vi "Arm Globals.vi"() -> ()   [LabVIEW 2012]
panel:
  in  "Arm Def Speed":dbl=0.5
  in  "Arm Dump Speed":dbl=1.0
  in  "Arm Dump Pos":dbl=90.0
  in  "Arm Mobile Pos":dbl=50.0
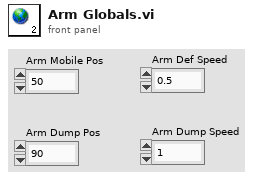
[diagram p1: front panel]
diagram:
